vi "recursive channel discovery.vi"(8 "error in (no error)":errorcluster, 11 "Controls[]":refnum<vi>[](array[refnum])) -> (0 "error out":errorcluster, 3 "Array":refnum<class "TBM channel.lvclass">[](array[class]))   [LabVIEW 2015, in "UI Reference configuration.lvclass"]
uses:
  UI Reference configuration.lvclass
  <vilib>/NI/Tag Bus Module Framework/channel/TBM channel.lvclass
  <vilib>/NI/Tag Bus Module Framework/channel/channel classification.ctl
  <vilib>/NI/Tag Bus/tag/Data Type.ctl
  <vilib>/Utility/VariantDataType/VariantType.lvlib
  <vilib>/NI/Tag Bus/tag/tag descriptor.lvclass
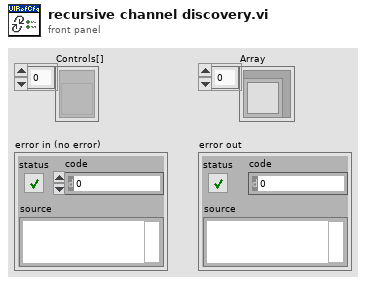
[diagram p1: front panel]
types:
  T1 = typedef "TBM channel.lvclass/channel classification.ctl" = enum16{"input data", "output data", "processing parameter", "processing result"}
  T2 = typedef "tag bus.lvlib/tag descriptor.lvclass/Data Type.ctl" = enum16{"Double", "Single", "I64", "I32", "I16", "I8", "U64", "U32", "U16", "U8", "Boolean", "String", "Array of Double", "Array of Single", "Array of I64", "Array of I32", "Array of I16", "Array of I8", "Array of U64", "Array of U32", "Array of U16", "Array of U8", "Array of Boolean", "Array of String"}
  T3 = typedef "VariantType.lvlib/Type.ctl" = enum8{"Invalid Type", "Void", "I8", "I16", "I32", "I64", "U8", "U16", "U32", "U64", "Single Float", "Double Float", "Extended Float", "Single Complex", "Double Complex", "Extended Complex", "Enum U8", "Enum U16", "Enum U32", "Enum U64", "Single Float With Unit", "Double Float With Unit", "Extended Float With Unit", "Single Complex with Unit", "Double Complex with Unit", "Extended Complex with Unit", "Boolean", "String", "Path", "Picture", "Tag", "Array", "Cluster", "Variant", "LV Variant", "Waveform", "Timestamp", "Digital Waveform", "Digital Data", "ExpressData", "Refnum", "External Data", "VI", "Poly VI", "LabVIEW Class Instance", "Fixed Point"}
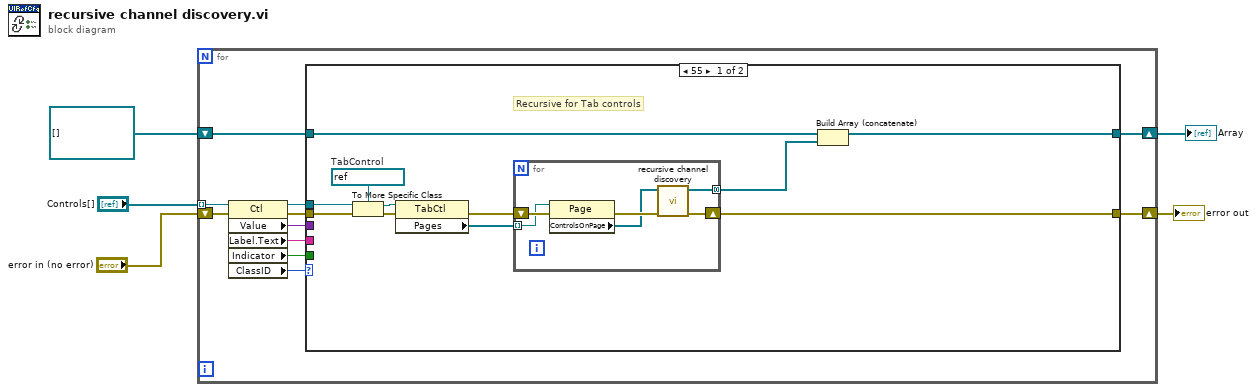
[diagram p0: block diagram]
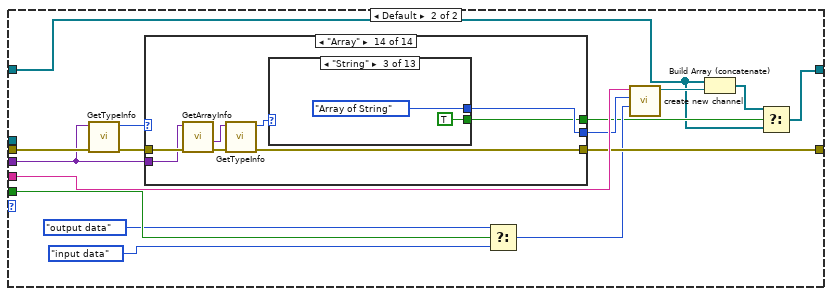
[diagram p2: hidden frame]
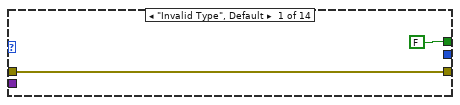
[diagram p3: hidden frame]
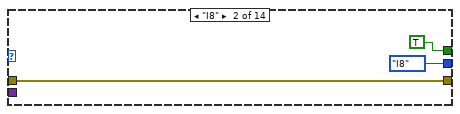
[diagram p4: hidden frame]
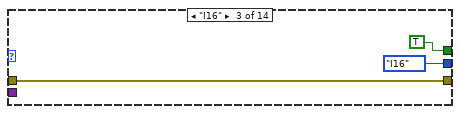
[diagram p5: hidden frame]
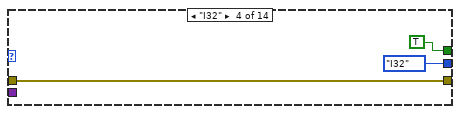
[diagram p6: hidden frame]
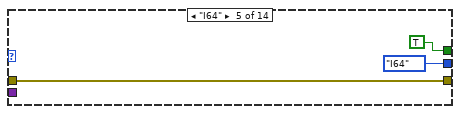
[diagram p7: hidden frame]
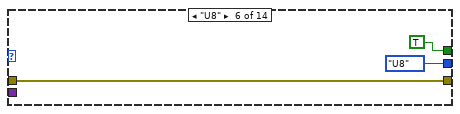
[diagram p8: hidden frame]
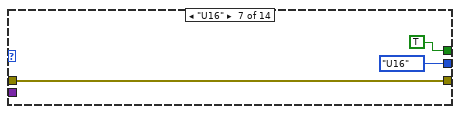
[diagram p9: hidden frame]
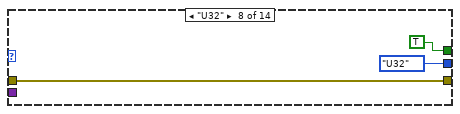
[diagram p10: hidden frame]
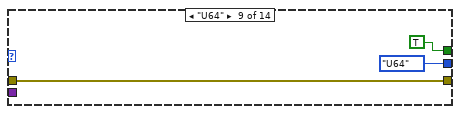
[diagram p11: hidden frame]
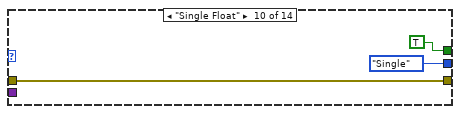
[diagram p12: hidden frame]
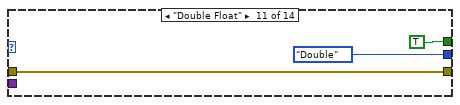
[diagram p13: hidden frame]
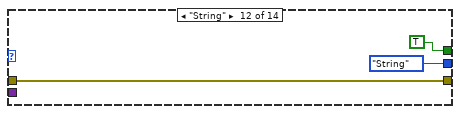
[diagram p14: hidden frame]
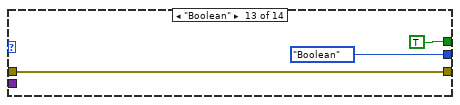
[diagram p15: hidden frame]
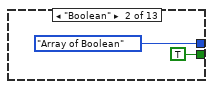
[diagram p17: hidden frame]
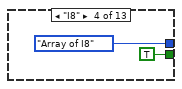
[diagram p18: hidden frame]
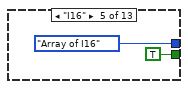
[diagram p19: hidden frame]
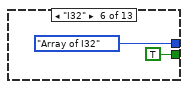
[diagram p20: hidden frame]
diagram:
  n1 = for {
    shift-right: [w10] -> w5
    shift-left: "error in (no error)" -> [w15]
    tunnel: "Controls[]" -> [w16] mode=indexing
    shift-right: [w6] -> w1
    shift-left: refnum<class "TBM channel.lvclass">[] [] ("Array") -> [w7]
    n2 = property class="Ctl"(reference=w16, error in=w15) -> (reference out=w8:refnum<vi>, error out=w12:errorcluster, "Value"=w11:variant, "Label.Text"=w14:string, "Indicator"=w13:bool, "ClassID"=w9:u32)
    n3 = case shown="55" w9 {
      tunnel: w14 -> [_ w49]
      tunnel: w13 -> [_ w48]
      tunnel: w12 -> [w27 w47]
      tunnel: w11 -> [_ w46]
      tunnel: [w17 w45] -> w10
      tunnel: w8 -> [w26 _]
      tunnel: w7 -> [w19 w34]
      tunnel: [w18 w35] -> w6
      frame 55 {
        w25 = refnum<vi> refnum  # TabControl
        # "Recursive for Tab controls"
        n4 = To More Specific Class(target class=w25, reference=w26, error in=w27) -> (specific class reference=w24:refnum<vi>, error out=w23:errorcluster)
        n5 = property class="TabCtl"(reference=w24, error in=w23) -> (error out=w21:errorcluster, "Pages"=w22:refnum<vi>[])  [unwired: 1 out]
        n6 = for {
          tunnel: w22 -> [w32] mode=indexing
          shift-right: [w29] -> w17
          shift-left: w21 -> [w33]
          tunnel: [w28] -> w20 mode=concatenating
          n7 = property class="Page"(reference=w32, error in=w33) -> (error out=w31:errorcluster, "ControlsOnPage"=w30:refnum<vi>[])  [unwired: 1 out]
          n8 = call "recursive channel discovery.vi"("error in (no error)"=w31, "Controls[]"=w30) -> ("error out"=w29:errorcluster, "Array"=w28:refnum<class "TBM channel.lvclass">[])  [unwired: 8 in]
        }
        n9 = Build Array (concatenate)(w19, w20) -> (w18:refnum<class "TBM channel.lvclass">[])
      }
      frame Default {
        n10 = call <vilib>:"GetTypeInfo.vi"("error in (no error)"=w47, "Variant"=w46) -> ("error out"=w40:errorcluster, "Type Enum"=w41:T3)  [unwired: 5 in, 3 out]
        n11 = case shown="\"Array\"" w41 {
          tunnel: w40 -> [w50 w52 w55 w58 w61 w64 w67 w70 w73 w76 w79 w82 w85 w95]
          tunnel: w46 -> [_ _ _ _ _ _ _ _ _ _ _ _ _ w94]
          tunnel: [FALSE TRUE TRUE TRUE TRUE TRUE TRUE TRUE TRUE TRUE TRUE TRUE TRUE w88] -> w38
          tunnel: [_ Data_Type."I8" ("data type") Data_Type."I16" ("data type") Data_Type."I32" ("data type") Data_Type."I64" ("data type") Data_Type."U8" ("data type") Data_Type."U16" ("data type") Data_Type."U32" ("data type") Data_Type."U64" ("data type") Data_Type."Single" ("data type") Data_Type."Double" ("data type") Data_Type."String" ("data type") Data_Type."Boolean" ("data type") w89] -> w39
          tunnel: [w50 w52 w55 w58 w61 w64 w67 w70 w73 w76 w79 w82 w85 w91] -> w45
          frame "Invalid Type", Default {
          }
          frame "I8" {
          }
          frame "I16" {
          }
          frame "I32" {
          }
          frame "I64" {
          }
          frame "U8" {
          }
          frame "U16" {
          }
          frame "U32" {
          }
          frame "U64" {
          }
          frame "Single Float" {
          }
          frame "Double Float" {
          }
          frame "String" {
          }
          frame "Boolean" {
          }
          frame "Array" {
            n12 = call <vilib>:"GetArrayInfo.vi"("error in (no error)"=w95, "Variant"=w94) -> ("error out"=w93:errorcluster, "ArrayElement"=w92:variant)  [unwired: 6 in, 2 out]
            n13 = call <vilib>:"GetTypeInfo.vi"("error in (no error)"=w93, "Variant"=w92) -> ("error out"=w91:errorcluster, "Type Enum"=w90:T3)  [unwired: 5 in, 3 out]
            n14 = case shown="\"String\"" w90 {
              tunnel: [_ Data_Type."Array of Boolean" ("data type") Data_Type."Array of String" ("data type") Data_Type."Array of I8" ("data type") Data_Type."Array of I16" ("data type") Data_Type."Array of I32" ("data type") Data_Type."Array of I64" ("data type") Data_Type."Array of U8" ("data type") Data_Type."Array of U16" ("data type") Data_Type."Array of U32" ("data type") Data_Type."Array of U64" ("data type") Data_Type."Array of Single" ("data type") Data_Type."Array of Double" ("data type")] -> w89
              tunnel: [_ TRUE TRUE TRUE TRUE TRUE TRUE TRUE TRUE TRUE TRUE TRUE TRUE] -> w88
              frame "Invalid Type", Default {
              }
              frame "Boolean" {
              }
              frame "String" {
              }
              frame "I8" {
              }
              frame "I16" {
              }
              frame "I32" {
              }
              frame "I64" {
              }
              frame "U8" {
              }
              frame "U16" {
              }
              frame "U32" {
              }
              frame "U64" {
              }
              frame "Single Float" {
              }
              frame "Double Float" {
              }
            }
          }
        }
        n15 = Select(t=channel_classification."output data" ("channel classification"), s=w48, f=channel_classification."input data" ("channel classification")) -> (s? t:f=w42:T1)
        n16 = call <vilib>:"create new channel.vi"("channel classification"=w42, "data type"=w39, "channel name"=w49) -> ("channel"=w37:refnum<class "TBM channel.lvclass">)  [unwired: 8 in]
        n17 = Build Array (concatenate)(w34, w37) -> (w36:refnum<class "TBM channel.lvclass">[])
        n18 = Select(t=w36, s=w38, f=w34) -> (s? t:f=w35:refnum<class "TBM channel.lvclass">[])
      }
    }
  }
  "Array" <- w1
  "error out" <- w5
